vi "2DarrayDBL-to-function.vi"(8 "error in (no error)":errorcluster caption="错误输入（无错误）", 9 "X":dbl, 10 "Y":dbl, 11 "2D array":dbl[][](array[numeric])) -> (0 "error out":errorcluster caption="错误输出", 1 "out-of-range":bool, 2 "f(x,y)":dbl)   [LabVIEW 2013]
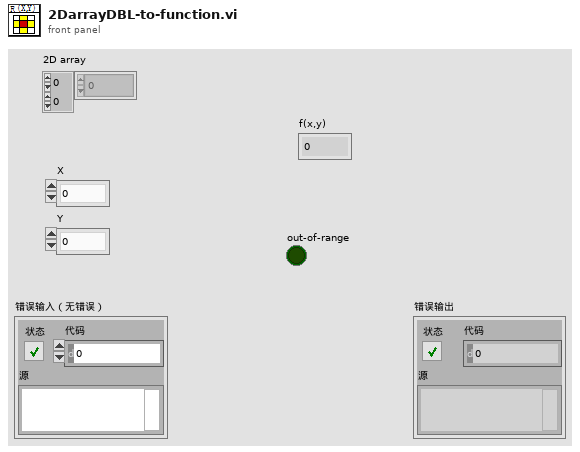
[diagram p1: front panel]
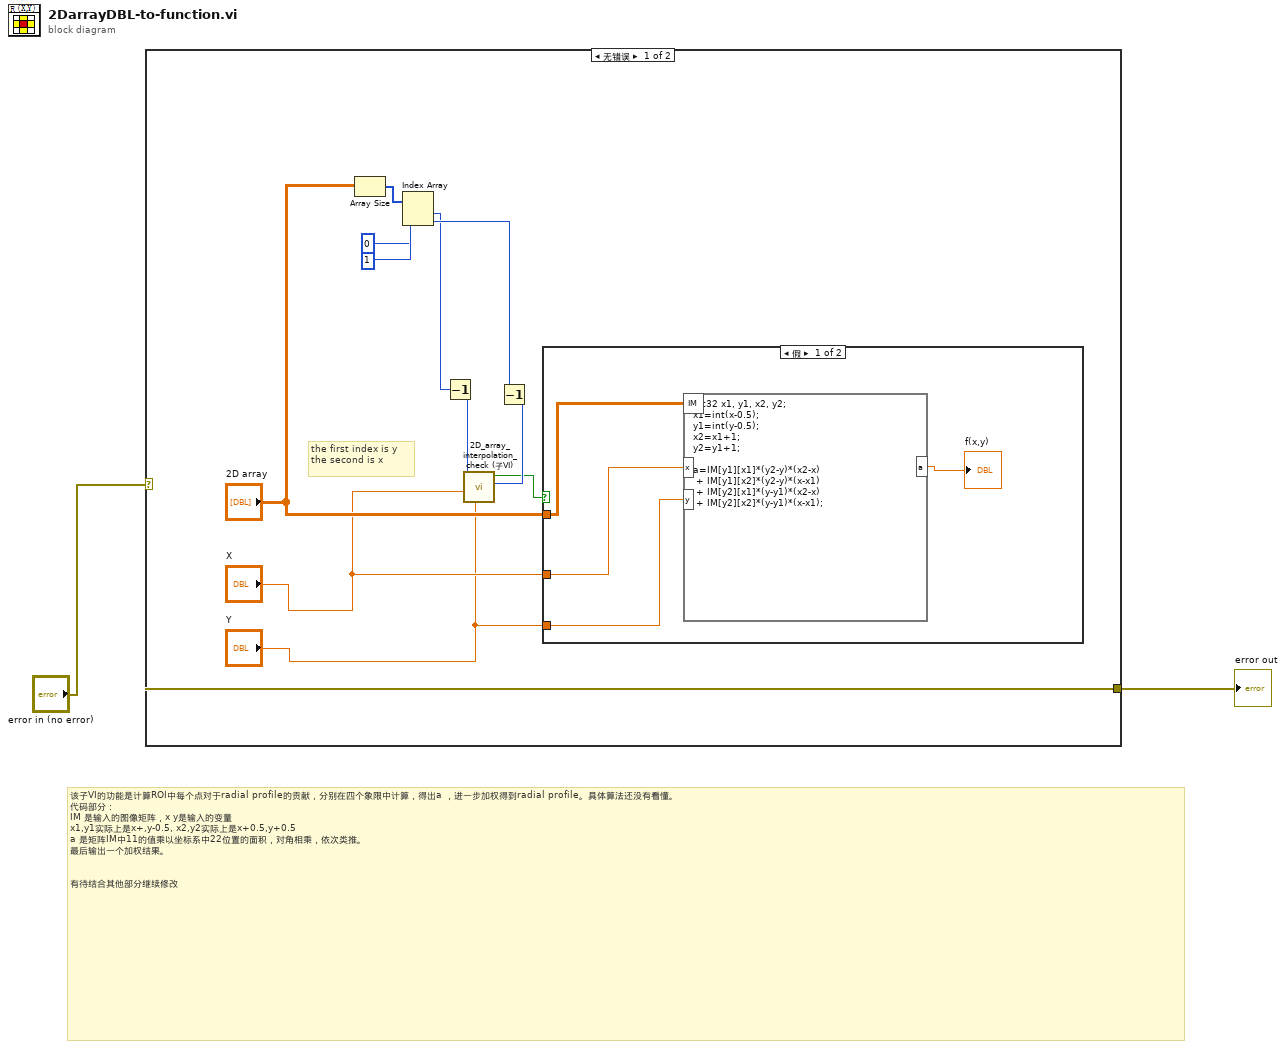
[diagram p0: block diagram]
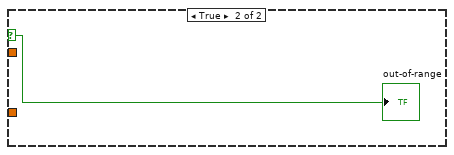
[diagram p2: hidden frame]
diagram:
  # "该子VI的功能是计算ROI中每个点对于radial profile的贡献，分别在四个象限中计算，得出a ，进一步加权得到radial profile。具体算法还没有看懂。\n代码部分：\nIM 是输入的图像矩阵，x y是输入的变量\nx1,y1实际上是x+,y-0.5, x2,y2实际上是x+0.5,y+0.5\na 是矩阵IM中11的值乘以坐标系中22位置的面积，对角相乘，依次类推。\n最后输出一个加权结果。\n\n\n有待结合其他部分继续修改"
  n1 = case shown="无错误" "error in (no error)" {
    selector: "error in (no error)" -> [w3 w20]
    tunnel: [w3 w20] -> w2
    frame No Error {
      # "the first index is y\nthe second is x"
      n2 = Array Size(array="2D array") -> (size(s)=w7:i32[])
      n3 = Index Array(array=w7, index #1=0 ("index"), index #2=1 ("index")) -> (element #1=w11:i32, element #2=w13:i32)
      n4 = Decrement(x=w11) -> (x-1=w12:i32)
      n5 = Decrement(x=w13) -> (x-1=w14:i32)
      n6 = call "2D_array_interpolation_check (子VI).vi"("yi"="Y", "xi"="X", "x信号个数"=w14, "y信号个数"=w12) -> ("布尔"=w6:bool)  [unwired: 7 in]
      n7 = case shown="假" w6 {
        selector: w6 -> [_ w19]
        tunnel: "2D array" -> [w17 _]
        tunnel: "X" -> [w16 _]
        tunnel: "Y" -> [w15 _]
        frame False {
          n8 = formula code="int32 x1, y1, x2, y2;\nx1=int(x-0.5);\ny1=int(y-0.5);\nx2=x1+1;\ny2=y1+1;\n\na=IM[y1][x1]*(y2-y)*(x2-x)\n + IM[y1][x2]*(y2-y)*(x-x1)\n + IM[y2][x1]*(y-y1)*(x2-x)\n + IM[y2][x2]*(y-y1)*(x-x1);"("x"=w16, "y"=w15, "IM"=w17) -> ("a"=→"f(x,y)":dbl)
        }
        frame True {
          "out-of-range" <- w19
        }
      }
    }
    frame Error {
    }
  }
  "error out" <- w2
